vi "_W_to_dBm.vi"(1 "Power W":dbl[](array[numeric])) -> (0 "Power dBm":dbl[](array[numeric]))   [LabVIEW 2013]
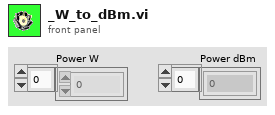
[diagram p1: front panel]
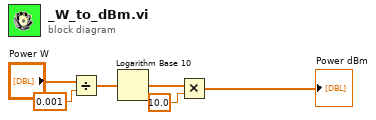
[diagram p0: block diagram]
diagram:
  n1 = Divide(x="Power W", y=0.001) -> (x/y=w3:dbl[])
  n2 = Logarithm Base 10(1:w3) -> (0:w4:dbl[])
  n3 = Multiply(x=w4, y=10.0) -> (x*y=→"Power dBm":dbl[])
